vi "通讯错误提示.vi"(11 "错误信息":string) -> (3 "重连？":bool)   [LabVIEW 2016]
panel:
  out "字符串":string
  in  "退出":bool
  in  "取消":bool
  in  "重连":bool
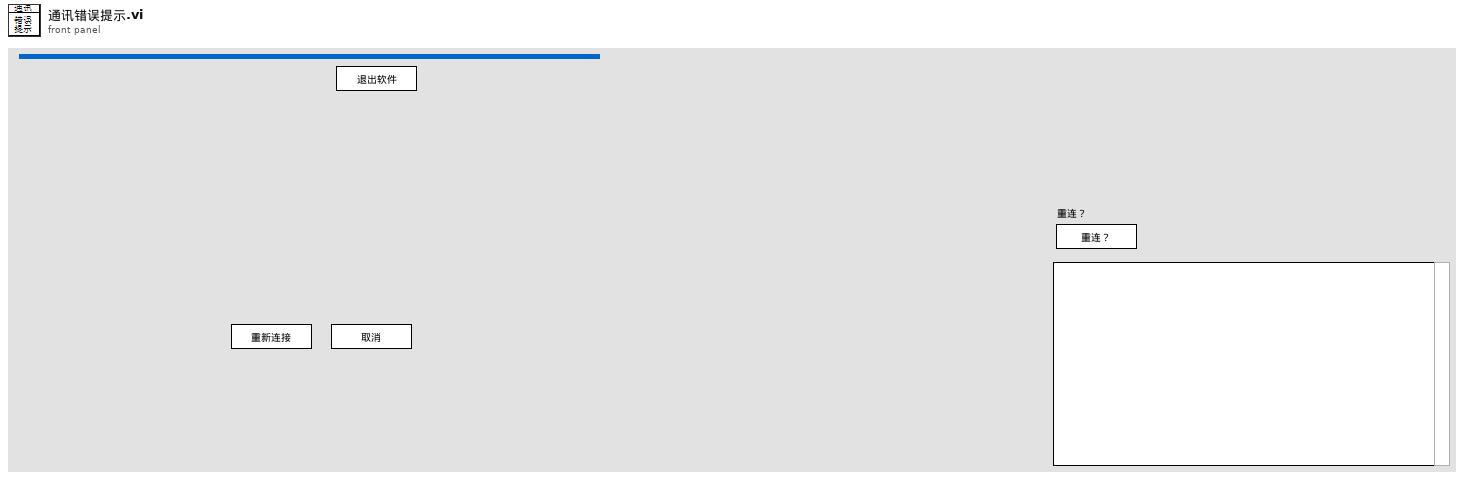
[diagram p1: front panel]
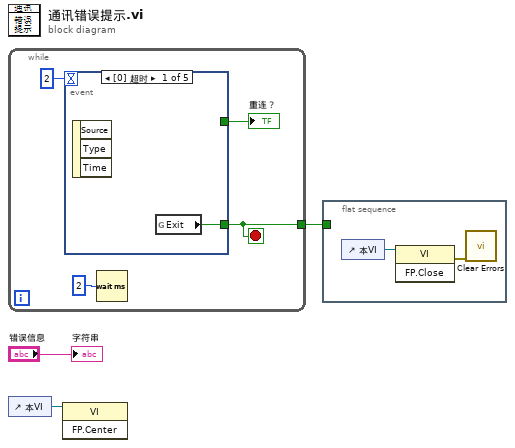
[diagram p0: block diagram]
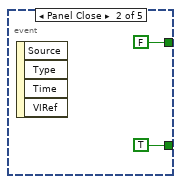
[diagram p2: hidden frame]
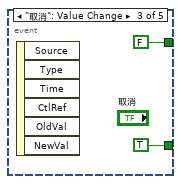
[diagram p3: hidden frame]
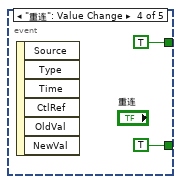
[diagram p4: hidden frame]
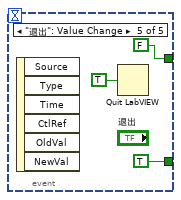
[diagram p5: hidden frame]
diagram:
  n1 = while {
    tunnel: [w5] -> w1
    stop <- w5 stop-if-true
    n2 = event shown="[0] 超时" {
      selector: _ -> [_ _ _ _ _]
      dyn-events: _ -> [_ _ _ _ _]
      timeout: 2 -> [_ _ _ _ _]
      tunnel: [w8 TRUE TRUE TRUE TRUE] -> w5
      tunnel: [_ FALSE FALSE TRUE FALSE] -> w7
      event Timeout {
        n3 = event-data() -> ()  [unwired: 1 in, 3 out]
        n4 = global read "全局.vi" "Exit"() -> (w8:bool)
      }
      event Panel Close {
        n5 = event-data() -> ()  [unwired: 1 in, 4 out]
      }
      event "取消": Value Change {
        n6 = event-data() -> ()  [unwired: 1 in, 6 out]
      }
      event "重连": Value Change {
        n7 = event-data() -> ()  [unwired: 1 in, 6 out]
      }
      event "退出": Value Change {
        n8 = event-data() -> ()  [unwired: 1 in, 6 out]
        n9 = Quit LabVIEW(quit? (T)=TRUE ("退出？(T)")) -> ()
      }
    }
    "重连？" <- w7
    n10 = Wait (ms)(milliseconds to wait=u32 2 ("等待时间（毫秒）")) -> ()  [unwired: 1 out]
  }
  n11 = control-ref of="本VI"() -> (w2:refnum<vi>)
  n12 = invoke class="VI" method="FP.Center"(reference=w2) -> ()  [unwired: 2 in, 3 out]
  n13 = flat-sequence {
    tunnel: w1 -> [_]
    frame #0 {
      n14 = control-ref of="本VI"() -> (w19:refnum<vi>)
      n15 = invoke class="VI" method="FP.Close"(reference=w19) -> (error out=w18:errorcluster)  [unwired: 2 in, 2 out]
      n16 = call <vilib>:"Clear Errors.vi"("error in (no error)"=w18) -> ()  [unwired: 5 in, 2 out]
    }
  }
  "字符串" <- "错误信息"
